vi "Sandbox.vi"() -> ()   [LabVIEW 2019]
panel:
  in  "Array 2":dbl[](array[numeric])=[0.0, 0.0, 0.0, 0.0]
  in  "Initialize":bool
  in  "Array":dbl[](array[numeric])=[0.0, 0.0, 0.0, 0.0]
  out "error out 2":errorcluster
  out "error out 5":errorcluster
  out "error out 6":errorcluster
  out "error out":errorcluster
  in  "Boolean":bool
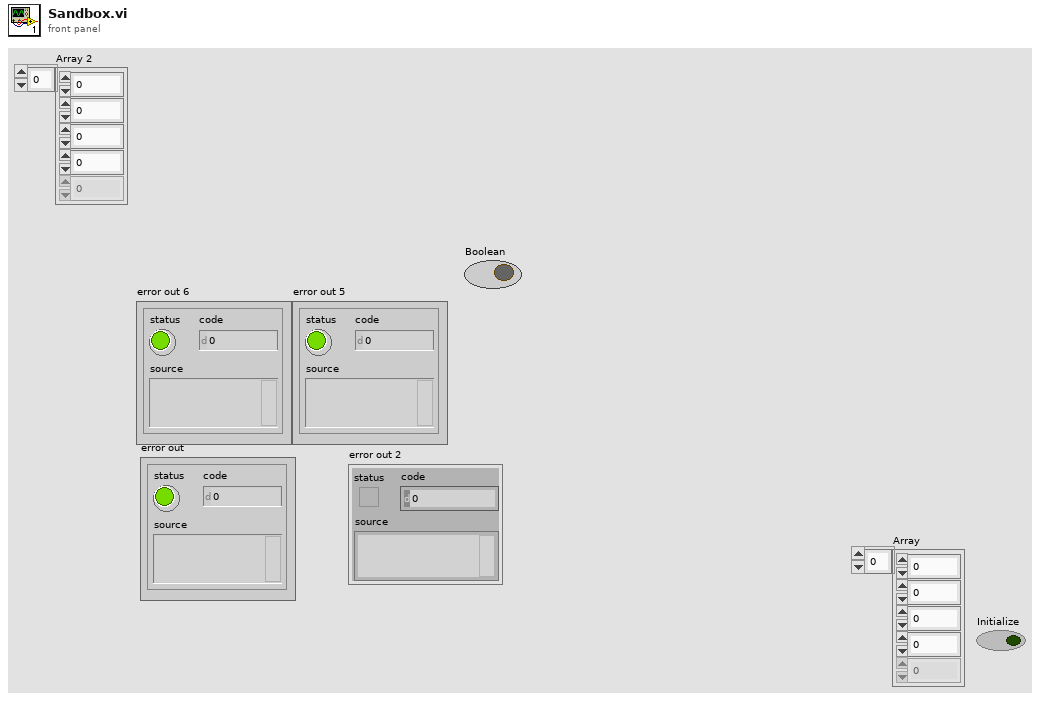
[diagram p1: front panel]
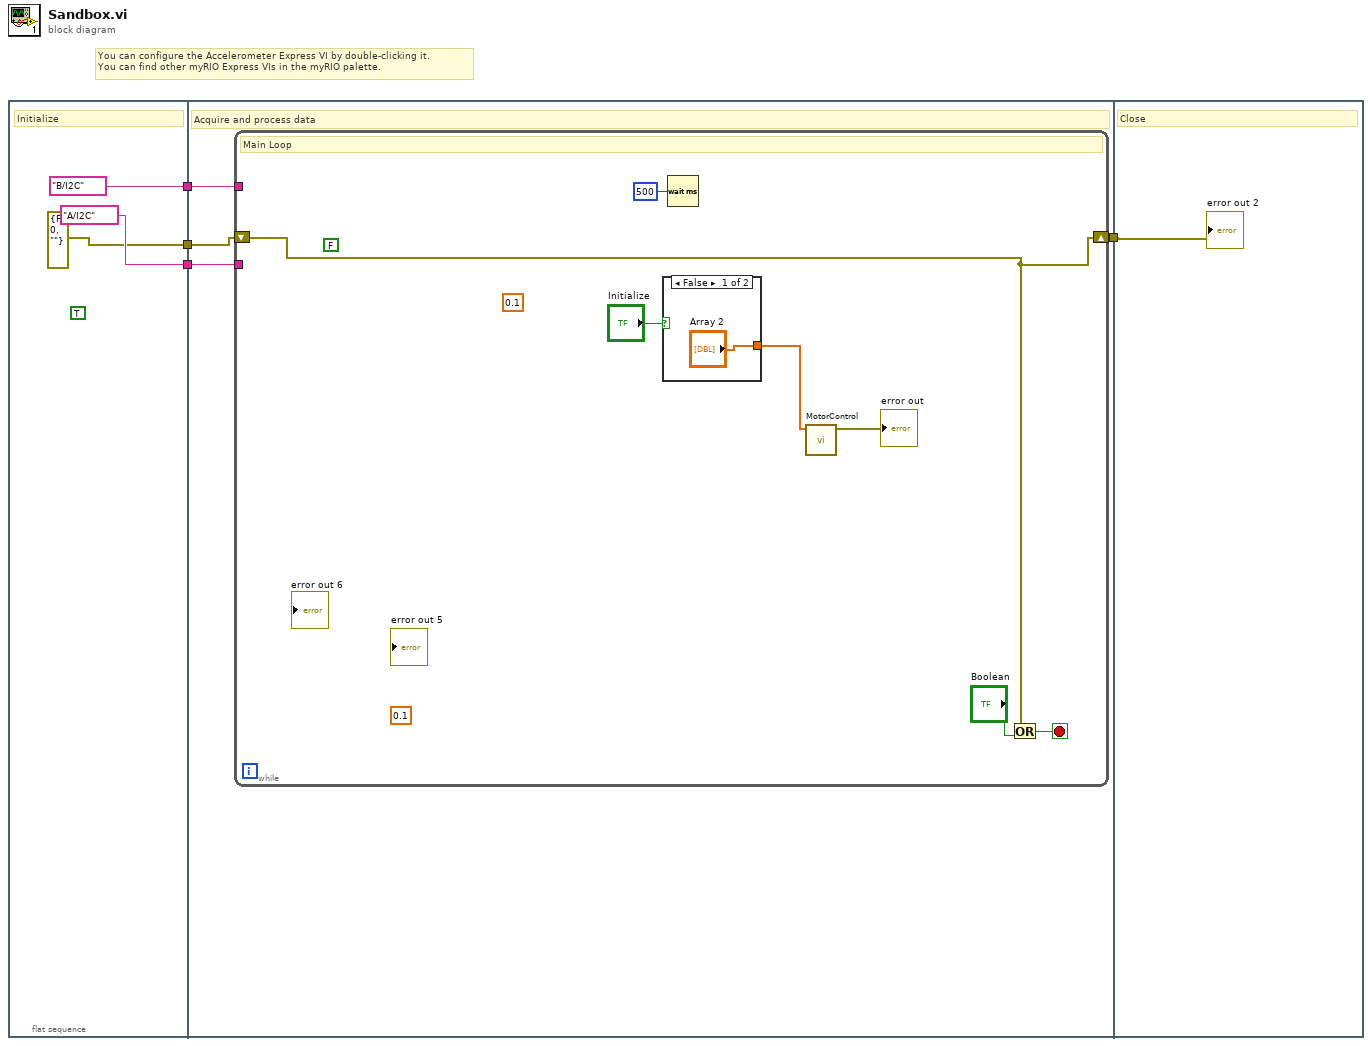
[diagram p0: block diagram]
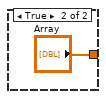
[diagram p2: hidden frame]
diagram:
  # "You can configure the Accelerometer Express VI by double-clicking it.\nYou can find other myRIO Express VIs in the myRIO palette."
  n1 = flat-sequence {
    tunnel: [tag "B/I2C" ("LIDAR Channel")] -> w4
    tunnel: [tag "A/I2C" ("IMU Channel")] -> w3
    tunnel: [errorcluster {"status"=FALSE, "code"=0, "source"=""} ("error in (no error)")] -> w2
    tunnel: [w11] -> w1
    tunnel: w4 -> [w10]
    tunnel: w3 -> [w9]
    tunnel: w2 -> [w8]
    tunnel: w1 -> [w21]
    frame #0 {
      (unwired) TRUE ("Calibrate?")
      # "Initialize"
    }
    frame #1 {
      # "Acquire and process data"
      n2 = while {
        shift-right: [w12] -> w11
        shift-left: w8 -> [w12]
        tunnel: w10 -> [_]
        tunnel: w9 -> [_]
        stop <- w18 stop-if-true
        (unwired) 0.1 ("low cutoff freq: fl")
        (unwired) 0.1 ("low cutoff freq: fl")
        (unwired) FALSE ("Calibrate?")
        # "Main Loop"
        n3 = case shown="False" "Initialize" {
          tunnel: ["Array 2" "Array"] -> w14
          frame False {
          }
          frame True {
          }
        }
        n4 = Wait (ms)(milliseconds to wait=u32 500) -> ()  [unwired: 1 out]
        n5 = call "MotorControl.vi"("Array"=w14) -> ("error out"=→"error out":errorcluster)  [unwired: 10 in]
        n6 = Or(x=w12, y="Boolean") -> (x .or. y?=w18:bool)
      }
    }
    frame #2 {
      # "Close"
      "error out 2" <- w21
    }
  }
